vi "Update Card Count.vi"(8 "new element/subarray":bool, 9 "cluster in":T1, 10 "# in":u32, 11 "Message Enqueuer":refnum<class "Message Enqueuer.lvclass">) -> (1 "cluster out":T1)   [LabVIEW 2013]
uses:
  <vilib>/ActorFramework/Message Enqueuer/Message Enqueuer.lvclass
  WT1600 Messages/Write Card Cluster Msg/Write Card Cluster Msg.lvclass/Write Card Cluster Msg.ctl
  <vilib>/ActorFramework/Message Enqueuer/Message Enqueuer.lvclass/Message Enqueuer.ctl
  <vilib>/ActorFramework/Message Enqueuer/Enqueue.vi
  <vilib>/ActorFramework/Message Priority Queue/Priority Enqueue.vi
  WT1600 Messages/Write Card Cluster Msg/Write Card Cluster Msg.lvclass
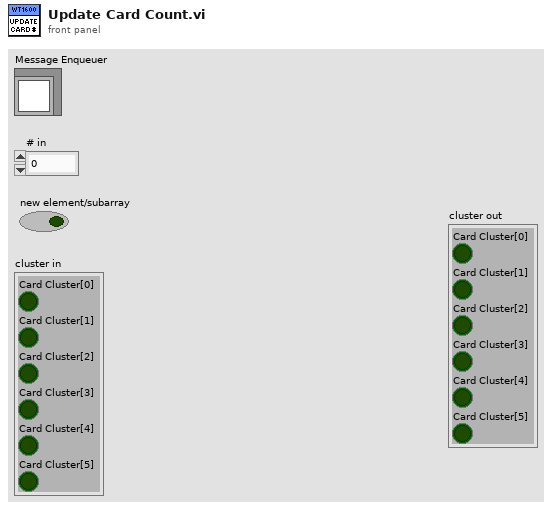
[diagram p1: front panel]
types:
  T1 = cluster{"Card Cluster[0]":bool, "Card Cluster[1]":bool, "Card Cluster[2]":bool, "Card Cluster[3]":bool, "Card Cluster[4]":bool, "Card Cluster[5]":bool}
  T2 = cluster{"cluster in[0]":bool, "cluster in[1]":bool, "cluster in[2]":bool, "cluster in[3]":bool, "cluster in[4]":bool, "cluster in[5]":bool}
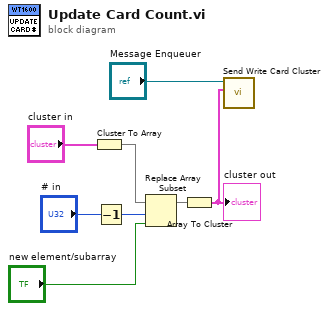
[diagram p0: block diagram]
diagram:
  n1 = Cluster To Array(cluster="cluster in") -> (array=w7:bool[])
  n2 = Decrement(x="# in") -> (x-1=w6:u32)
  n3 = Replace Array Subset(array=w7, new element="new element/subarray", index=w6) -> (w5:bool[])
  n4 = Array To Cluster(array=w5) -> (cluster=w2:T2)
  "cluster out" <- w2
  n5 = call "Send Write Card Cluster.vi"("Card Cluster"=w2, "Message Enqueuer"="Message Enqueuer") -> ()  [unwired: 8 in, 2 out]
